vi "Generate report.vi"(11 "Queues":T1) -> ()   [LabVIEW 2014]
uses:
  CMD UI enum.ctl
  CMD Report enum.ctl
  CMD DA enum.ctl
  CMD DAQ enum.ctl
  CMD LOG enum.ctl
  patiant and daq params.ctl
  set_get.ctl
  <vilib>/Utility/NIReport.llb/Append Report Text (str wrap).vi
  <vilib>/Utility/NIReport.llb/Append Text Table to Report (wrap).vi
  <vilib>/Utility/NIReport.llb/NI_report.lvclass
panel:
  out "error out":errorcluster
  in  "Patient Name":string
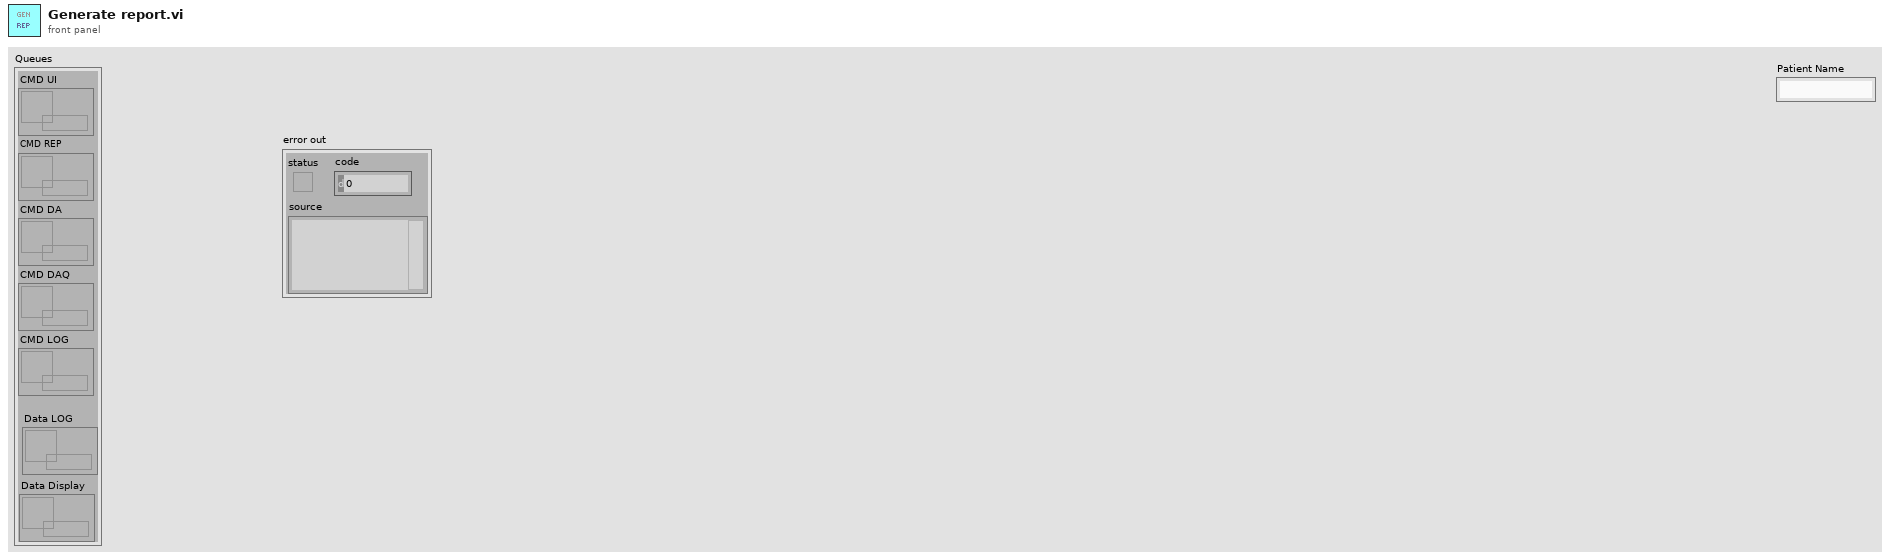
[diagram p1: front panel]
types:
  T1 = cluster{"CMD UI":refnum<queue>, "CMD REP":refnum<queue>, "CMD DA":refnum<queue>, "CMD DAQ":refnum<queue>, "CMD LOG":refnum<queue>, "Data LOG":refnum<queue>, "Data Display":refnum<queue>}
  T2 = cluster{"position (excel)":cluster{"row":i32, "column":i32}, "name (excel)":string, "bookmark (word)":string}
  T3 = typedef "set_get.ctl" = enum16{"Set", "Get"}
  T4 = typedef "patiant and daq params.ctl" = cluster{"DAQ Parameters":cluster{"Sampling rate":dbl, "Max_volt":dbl, "Min_volt":dbl, "DAQmx Physical Channels \nHR,SC":tag, "Resting State":bool, "Analyze every (s)":dbl}, "Patient Info \n(Updates automatically when reading from file)":cluster{"Patient Name":string, "Patient ID":string, "Patient Age":dbl, "Gender":string}, "Raw Data Read Path":path, "Avg HR ":dbl, "Avg SC  ":dbl}
  T5 = cluster{"The Cluster":T4, "Arterial Pressure (Raw Data)":refnum<vi>, "Skin Conductance (Raw Data)":refnum<vi>, "HR":refnum<vi>, "Skin Conductance":refnum<vi>}
  T6 = enum16{"Standard Report", "HTML", "Word", "Excel"}
  T7 = typedef "CMD Report enum.ctl" = enum16{"Create Report", "Exit"}
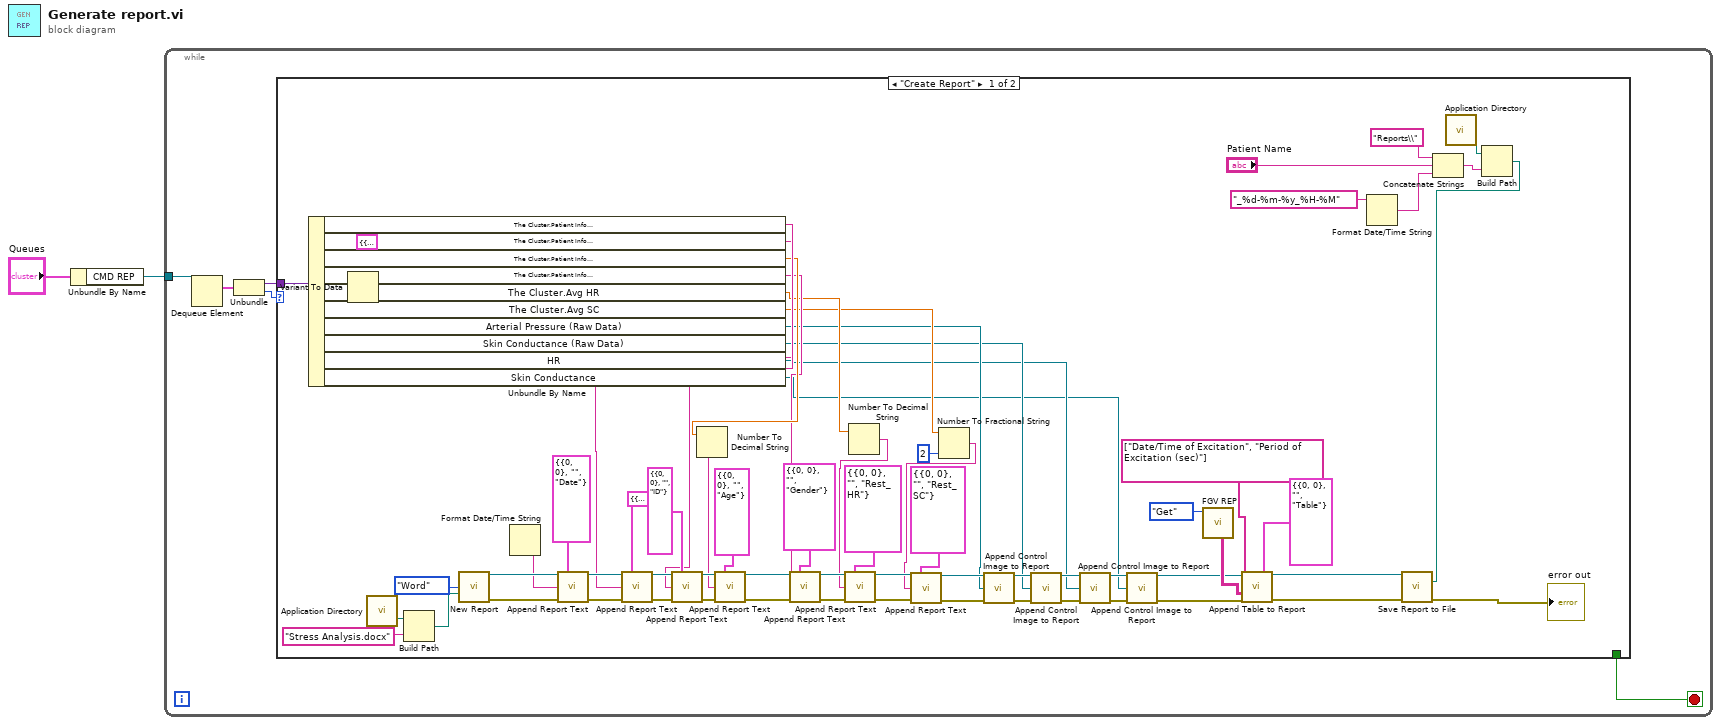
[diagram p0: block diagram]
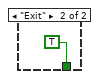
[diagram p2: hidden frame]
diagram:
  n1 = Unbundle By Name("Queues") -> ("CMD REP"=w1:refnum<queue>)
  n2 = while {
    tunnel: w1 -> [w3]
    stop <- w5 stop-if-true
    n3 = Dequeue Element(queue=w3) -> (element=w7:cluster{variant, T7})  [unwired: 2 in, 3 out]
    n4 = Unbundle(w7) -> (w4:variant, w6:T7)
    n5 = case shown="\"Create Report\"" w6 {
      tunnel: [_ TRUE] -> w5
      tunnel: w4 -> [w58 _]
      frame "Create Report" {
        n6 = Variant To Data(type=T5 {"The Cluster"={"DAQ Parameters"={"Sampling rate"=0.0, "Max_volt"=0.0, "Min_volt"=0.0, "DAQmx Physical Channels \nHR,SC"="", "Resting State"=FALSE, "Analyze every (s)"=0.0}, "Patient Info \n(Updates automatically when reading from file)"={"Patient Name"="", "Patient ID"="", "Patient Age"=0.0, "Gender"=""}, "Raw Data Read Path"=path "", "Avg HR "=0.0, "Avg SC  "=0.0}, "Arterial Pressure (Raw Data)"=refnum, "Skin Conductance (Raw Data)"=refnum, "HR"=refnum, "Skin Conductance"=refnum} ("output cluster"), Variant=w58) -> (data=w56:T5)  [unwired: 1 in, 1 out]
        n7 = Unbundle By Name(w56) -> ("The Cluster.Patient Info \n(Updates automatically when reading from file).Patient Name"=w50:string, "The Cluster.Patient Info \n(Updates automatically when reading from file).Patient ID"=w49:string, "The Cluster.Patient Info \n(Updates automatically when reading from file).Patient Age"=w46:dbl, "The Cluster.Patient Info \n(Updates automatically when reading from file).Gender"=w40:string, "The Cluster.Avg HR"=w35:dbl, "The Cluster.Avg SC"=w29:dbl, "Arterial Pressure (Raw Data)"=w20:refnum<vi>, "Skin Conductance (Raw Data)"=w19:refnum<vi>, "HR"=w18:refnum<vi>, "Skin Conductance"=w17:refnum<vi>)
        n8 = call <vilib>:"Application Directory.vi"() -> ("Application Directory"=w72:path)
        n9 = Build Path(base path=w72, name or relative path="Stress Analysis.docx") -> (appended path=w73:path)
        n10 = call <vilib>:"New Report.vi"("report type"=T6."Word", "template (empty)"=w73) -> ("report out"=w62:refnum<class "NI_report.lvclass">, "error out"=w61:errorcluster)  [unwired: 12 in]
        n11 = Format Date/Time String() -> (date/time string=w60:string)  [unwired: 3 in]
        n12 = call-poly <vilib>:"Append Report Text.vi"("report in"=w62, "MS Office parameters"=T2 {"position (excel)"={"row"=0, "column"=0}, "name (excel)"="", "bookmark (word)"="Date"}, "text"=w60, "error in (no error)"=w61) -> ("report out"=w63:refnum<class "NI_report.lvclass">, "error out"=w55:errorcluster)  [unwired: 8 in, 2 out]
        n13 = call-poly <vilib>:"Append Report Text.vi"("report in"=w63, "MS Office parameters"=T2 {"position (excel)"={"row"=0, "column"=0}, "name (excel)"="", "bookmark (word)"="Name"}, "text"=w50, "error in (no error)"=w55) -> ("report out"=w53:refnum<class "NI_report.lvclass">, "error out"=w52:errorcluster)  [unwired: 8 in, 2 out]
        n14 = call-poly <vilib>:"Append Report Text.vi"("report in"=w53, "MS Office parameters"=T2 {"position (excel)"={"row"=0, "column"=0}, "name (excel)"="", "bookmark (word)"="ID"}, "text"=w49, "error in (no error)"=w52) -> ("report out"=w48:refnum<class "NI_report.lvclass">, "error out"=w47:errorcluster)  [unwired: 8 in, 2 out]
        n15 = Number To Decimal String(number=w46) -> (decimal integer string=w45:string)  [unwired: 1 in]
        n16 = call-poly <vilib>:"Append Report Text.vi"("report in"=w48, "MS Office parameters"=T2 {"position (excel)"={"row"=0, "column"=0}, "name (excel)"="", "bookmark (word)"="Age"}, "text"=w45, "error in (no error)"=w47) -> ("report out"=w43:refnum<class "NI_report.lvclass">, "error out"=w42:errorcluster)  [unwired: 8 in, 2 out]
        n17 = call-poly <vilib>:"Append Report Text.vi"("report in"=w43, "MS Office parameters"=T2 {"position (excel)"={"row"=0, "column"=0}, "name (excel)"="", "bookmark (word)"="Gender"}, "text"=w40, "error in (no error)"=w42) -> ("report out"=w39:refnum<class "NI_report.lvclass">, "error out"=w38:errorcluster)  [unwired: 8 in, 2 out]
        n18 = Number To Decimal String(number=w35) -> (decimal integer string=w36:string)  [unwired: 1 in]
        n19 = call-poly <vilib>:"Append Report Text.vi"("report in"=w39, "MS Office parameters"=T2 {"position (excel)"={"row"=0, "column"=0}, "name (excel)"="", "bookmark (word)"="Rest_HR"}, "text"=w36, "error in (no error)"=w38) -> ("report out"=w32:refnum<class "NI_report.lvclass">, "error out"=w31:errorcluster)  [unwired: 8 in, 2 out]
        n20 = Number To Fractional String(number=w29, precision (6)=i16 2) -> (F-format string=w30:string)  [unwired: 2 in]
        n21 = call-poly <vilib>:"Append Report Text.vi"("report in"=w32, "MS Office parameters"=T2 {"position (excel)"={"row"=0, "column"=0}, "name (excel)"="", "bookmark (word)"="Rest_SC"}, "text"=w30, "error in (no error)"=w31) -> ("report out"=w26:refnum<class "NI_report.lvclass">, "error out"=w25:errorcluster)  [unwired: 8 in, 2 out]
        n22 = call-dynamic "Append Control Image to Report.vi"("report in"=w26, "ctrl reference"=w20, "error in (no error)"=w25) -> ("report out"=w28:refnum<class "NI_report.lvclass">, "error out"=w27:errorcluster)  [unwired: 9 in, 2 out]
        n23 = call-dynamic "Append Control Image to Report.vi"("report in"=w28, "ctrl reference"=w19, "error in (no error)"=w27) -> ("report out"=w22:refnum<class "NI_report.lvclass">, "error out"=w21:errorcluster)  [unwired: 9 in, 2 out]
        n24 = call-dynamic "Append Control Image to Report.vi"("report in"=w22, "ctrl reference"=w18, "error in (no error)"=w21) -> ("report out"=w23:refnum<class "NI_report.lvclass">, "error out"=w24:errorcluster)  [unwired: 9 in, 2 out]
        n25 = call-dynamic "Append Control Image to Report.vi"("report in"=w23, "ctrl reference"=w17, "error in (no error)"=w24) -> ("report out"=w13:refnum<class "NI_report.lvclass">, "error out"=w12:errorcluster)  [unwired: 9 in, 2 out]
        n26 = call "FGV REP.vi"("Enum"=set_get."Get") -> ("Array"=w15:string[][])  [unwired: 10 in]
        n27 = call-poly <vilib>:"Append Table to Report.vi"("report in"=w13, "MS Office parameters"=T2 {"position (excel)"={"row"=0, "column"=0}, "name (excel)"="", "bookmark (word)"="Table"}, "column headers"=string[] ["Date/Time of Excitation", "Period of Excitation (sec)"], "text data"=w15, "error in (no error)"=w12) -> ("report out"=w10:refnum<class "NI_report.lvclass">, "error out"=w9:errorcluster)  [unwired: 7 in, 2 out]
        n28 = Format Date/Time String(time format string (%c)="_%d-%m-%y_%H-%M") -> (date/time string=w66:string)  [unwired: 2 in]
        n29 = Concatenate Strings("Reports\\" ("string"), "Patient Name", w66) -> (w68:string)
        n30 = call <vilib>:"Application Directory.vi"() -> ("Application Directory"=w69:path)
        n31 = Build Path(base path=w69, name or relative path=w68) -> (appended path=w64:path)
        n32 = call-dynamic "Save Report to File.vi"("report in"=w10, "report file path"=w64, "error in (no error)"=w9) -> ("error out"=→"error out":errorcluster)  [unwired: 11 in, 1 out]
      }
      frame "Exit" {
      }
    }
  }
